vi "Scan_Frequency_Range.vi"() -> ()   [LabVIEW 2010]
uses:
  <vilib>/Utility/file.llb/Write To Spreadsheet File (DBL).vi
panel:
  in  "Step size":dbl=1.0
  in  "Max. Frequency":dbl=20.0
  in  "Wait":dbl=1.0
  in  "Path":path
  out "XY Graph 2":cluster{dbl[], dbl[]}(graph)
  out "error out":errorcluster
  in  "error in (no error)":errorcluster
  out "atStep":dbl format="%.2f"
  in  "Start":dbl format="%.2f"
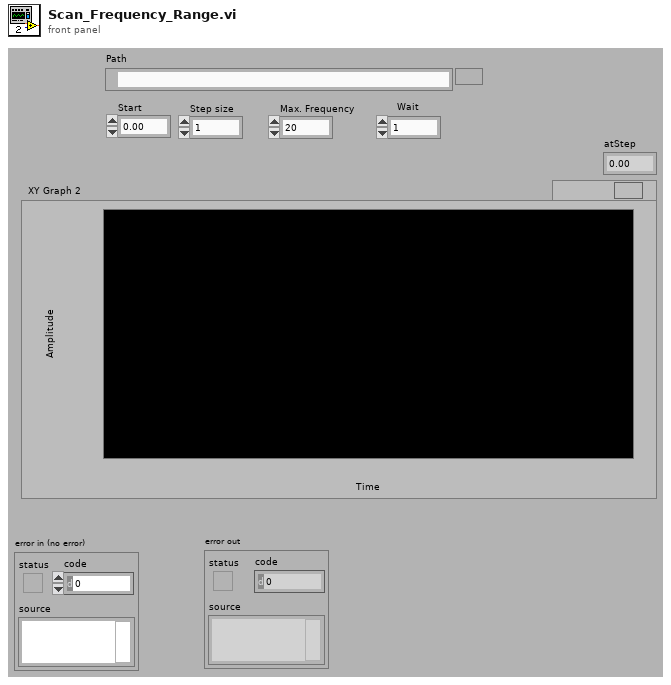
[diagram p1: front panel]
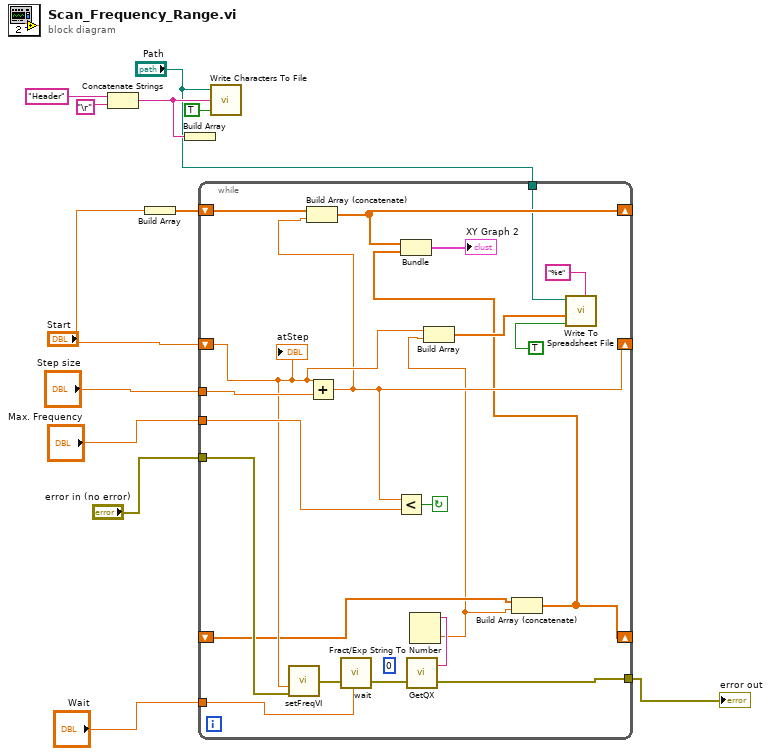
[diagram p0: block diagram]
diagram:
  n1 = Concatenate Strings("Header", "\r") -> (w5:string)
  n2 = Build Array("Start") -> (w9:dbl[])
  n3 = Build Array(w5) -> ()  [unwired: 1 out]
  n4 = while {
    tunnel: "error in (no error)" -> [w25]
    tunnel: [w22] -> w11
    shift-right: [w16] -> _
    shift-left: "Start" -> [w17]
    shift-right: [w20] -> _
    shift-left: w9 -> [w32]
    tunnel: "Path" -> [w18]
    tunnel: "Wait" -> [w27]
    tunnel: "Max. Frequency" -> [w26]
    tunnel: "Step size" -> [w19]
    shift-right: [w13] -> _
    shift-left: _ -> [w15]
    stop <- w33 continue-if-true
    (unwired) 0
    n5 = call "setFreqVI.vi"("error in"=w25, "Frequenz in Hz"=w17) -> ("error out"=w24:errorcluster)  [unwired: 2 in]
    n6 = Add(x=w17, y=w19) -> (x+y=w16:dbl)
    n7 = Build Array (concatenate)(w32, w16) -> (w20:dbl[])
    n8 = call "wait.vi"("error in"=w24, "Wartezeit in Sek"=w27) -> ("error out"=w23:errorcluster)  [unwired: 1 in]
    n9 = Less?(x=w16, y=w26) -> (x < y?=w33:bool)
    n10 = call "GetQX.vi"("error in"=w23) -> ("error out"=w22:errorcluster, "data"=w21:string)  [unwired: 1 in]
    n11 = Fract/Exp String To Number(string=w21) -> (number=w14:dbl)  [unwired: 3 in, 1 out]
    n12 = Build Array(w17, w14) -> (w28:dbl[])
    n13 = Build Array (concatenate)(w15, w14) -> (w13:dbl[])
    n14 = Bundle(w20, w13) -> (→"XY Graph 2":cluster{dbl[], dbl[]})  [unwired: 1 in]
    n15 = call-poly <vilib>:"Write To Spreadsheet File.vi"("format (%.3f)"="%e", "append to file? (new file:F)"=TRUE, "1D data"=w28, "file path (dialog if empty)"=w18) -> ()  [unwired: 4 in, 1 out]
    "atStep" <- w17
  }
  "error out" <- w11
  n16 = call <vilib>:"Write Characters To File.vi"("append to file? (new file:F)"=TRUE, "character string"=w5, "file path (dialog if empty)"="Path") -> ()  [unwired: 2 in, 1 out]
